vi "Template update scenario templates.vi"(8 "error in (no error)":errorcluster, 9 "ixTemplate (0)":i32, 10 "new name":string, 11 "Connection Refnum":T1) -> (0 "error out":errorcluster, 3 "Connection Refnum":T1)   [LabVIEW 2011]
uses:
  SI.LIB/ODBC/SQL Controls/Connection Refnum.ctl
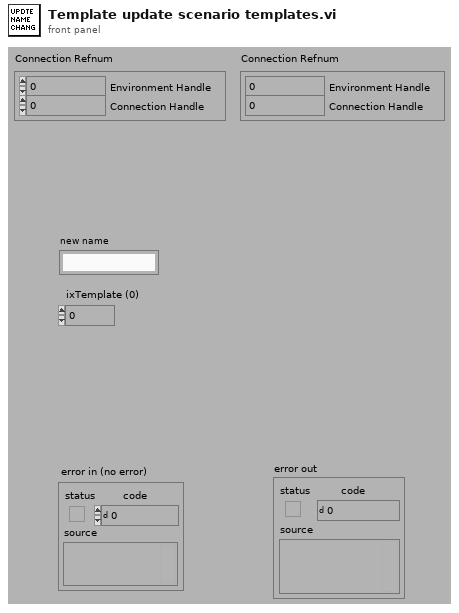
[diagram p1: front panel]
types:
  T1 = typedef "Connection Refnum.ctl" = cluster{"Environment Handle":i32, "Connection Handle":i32}
  T2 = typedef "Template Record.ctl" = cluster{"ixTemplate":i32, "sxTemplateId":string, "sDescription":string, "sCreator":string, "tCreationDate":timestamp, "sModifier":string, "tModifiedDate":timestamp, "sType":string, "sStyle":string, "sFormat":string, "dWidth":dbl, "dHeight":dbl, "sFilename":string, "sScript":string, "sLayout":string, "sEditor":string, "sStyleProcess":string}
  T3 = typedef "Scenario Record.ctl" = cluster{"ixScenario":i32, "tCreated":timestamp, "tModified":timestamp, "sxUsername":string, "sModifiedBy":string, "sxScenarioId":string, "sDescription":string, "sLogic":string, "sResultFieldsCSV":string, "sTemplatesCSV":string, "fAutoRunReports":bool, "fSortByTemplates":bool, "fCombinePDF":bool, "Conditions":T4[]}
  T4 = typedef "Condition Record.ctl" = cluster{"iConditionIndex":i32, "sxFieldId":string, "nOperator":T5, "sMatchValue":string}
  T5 = typedef "Condition Operators.ctl" = enum16{"equal (=)", "not equal (\\u2260)", "less than (<)", "less than or equal (\\u2264)", "greater than (>)", "greater than or equal (\\u2265)", "contains", "does not contain"}
  T6 = typedef "Step Record.ctl" = cluster{"ixStep":i32, "sxSequenceId":string, "sxTestId":string, "iIndex":i32, "iRepeat":i32, "iQuickMode":i32, "sTag":string, "sDatasheetsCSV":string, "bConfiguration":string}
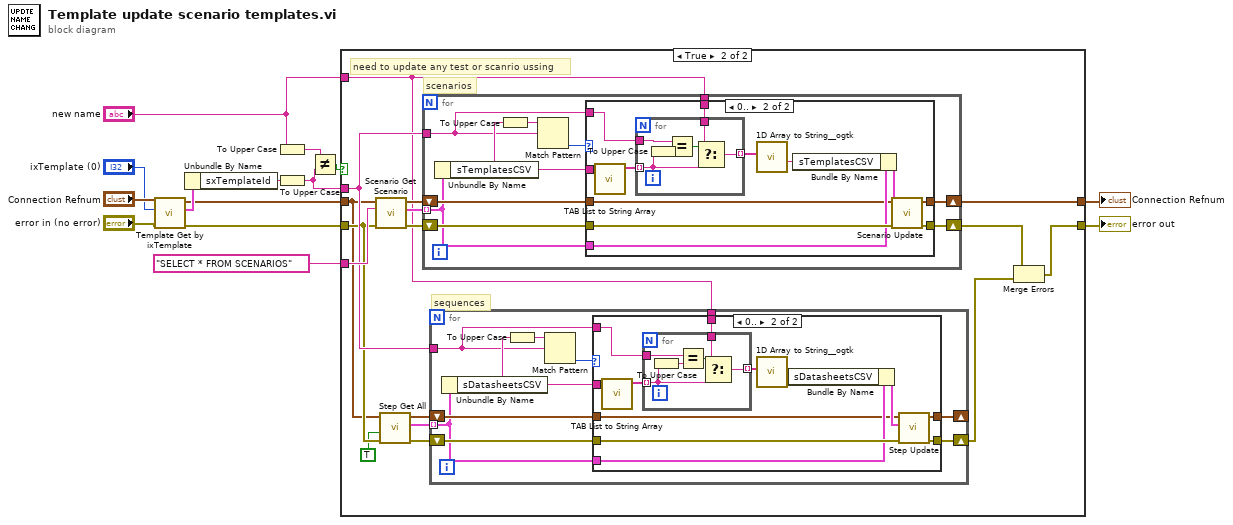
[diagram p0: block diagram]
diagram:
  n1 = call "Template Get by ixTemplate.vi"("error in (no error)"="error in (no error)", "ixTemplate (0)"="ixTemplate (0)", "Connection Refnum"="Connection Refnum") -> ("error out"=w8:errorcluster, "Template Record"=w14:T2, "Connection Refnum"=w6:T1)  [unwired: 6 out]
  n2 = Unbundle By Name(w14) -> ("sxTemplateId"=w13:string)
  n3 = To Upper Case(1:"new name") -> (0:w3:string)
  n4 = To Upper Case(1:w13) -> (0:w2:string)
  n5 = Not Equal?(x=w3, y=w2) -> (x != y?=w9:bool)
  n6 = case shown="True" w9 {
    tunnel: w8 -> [w16 w26]
    tunnel: [w16 w18] -> w7
    tunnel: w6 -> [w15 w21]
    tunnel: [w15 w28] -> w5
    tunnel: "SELECT * FROM SCENARIOS" -> [_ w32]
    tunnel: w2 -> [_ w27]
    tunnel: "new name" -> [_ w22]
    frame False {
      # "same name no update needed"
    }
    frame True {
      # "sequences"
      # "scenarios"
      # "need to update any test or scanrio ussing"
      n7 = call "Scenario Get Scenario.vi"("error in (no error)"=w26, "Query"=w32, "Connection Refnum"=w21) -> ("error out"=w30:errorcluster, "Scenarios"=w31:T3[], "Connection Refnum"=w29:T1)  [unwired: 6 out]
      n8 = call "Step Get All.vi"("error in (no error)"=w26, "All Steps? (f)"=TRUE, "Connection Refnum"=w21) -> ("error out"=w23:errorcluster, "Sequence Steps"=w24:T6[], "Connection Refnum"=w25:T1)  [unwired: 1 in, 5 out]
      n9 = for {
        tunnel: w31 -> [w65] mode=indexing
        shift-right: [w68] -> w20
        shift-left: w30 -> [w69]
        shift-right: [w66] -> w28
        shift-left: w29 -> [w67]
        tunnel: w27 -> [w64]
        tunnel: w22 -> [w63]
        n10 = Unbundle By Name(w65) -> ("sTemplatesCSV"=w72:string)
        n11 = To Upper Case(1:w72) -> (0:w71:string)
        n12 = Match Pattern(string=w71, regular expression=w64) -> (offset past match=w70:i32)  [unwired: 4 out]
        n13 = case shown="0.." w70 {
          tunnel: w72 -> [_ w86]
          tunnel: w69 -> [w74 w85]
          tunnel: [w74 w84] -> w68
          tunnel: w67 -> [w73 w80]
          tunnel: [w73 w83] -> w66
          tunnel: w65 -> [_ w82]
          tunnel: w64 -> [_ w78]
          tunnel: w63 -> [_ w77]
          frame Default {
          }
          frame 0.. {
            n14 = call "TAB List to String Array.vi"("String"=w86) -> ("Array"=w79:string[])  [unwired: 10 out]
            n15 = for {
              tunnel: w79 -> [w90] mode=indexing
              tunnel: w78 -> [w91]
              tunnel: [w89] -> w76 mode=indexing
              tunnel: w77 -> [w88]
              n16 = To Upper Case(1:w90) -> (0:w87:string)
              n17 = Equal?(x=w91, y=w87) -> (x = y?=w92:bool)
              n18 = Select(t=w88, s=w92, f=w90) -> (s? t:f=w89:string)
            }
            n19 = call "1D Array to String__ogtk.vi"("Array of Strings"=w76) -> ("delimited string"=w75:string)  [unwired: 10 in]
            n20 = Bundle By Name(cluster=w82, "sTemplatesCSV"=w75) -> (w81:T3)
            n21 = call "Scenario Update.vi"("error in (no error)"=w85, "Scenario (none)"=w81, "Connection Refnum"=w80) -> ("error out"=w84:errorcluster, "Connection Refnum"=w83:T1)  [unwired: 7 out]
          }
        }
      }
      n22 = for {
        tunnel: w24 -> [w35] mode=indexing
        shift-right: [w38] -> w19
        shift-left: w23 -> [w39]
        shift-right: [w36] -> _
        shift-left: w25 -> [w37]
        tunnel: w27 -> [w34]
        tunnel: w22 -> [w33]
        n23 = Unbundle By Name(w35) -> ("sDatasheetsCSV"=w42:string)
        n24 = To Upper Case(1:w42) -> (0:w41:string)
        n25 = Match Pattern(string=w41, regular expression=w34) -> (offset past match=w40:i32)  [unwired: 4 out]
        n26 = case shown="0.." w40 {
          tunnel: w42 -> [_ w56]
          tunnel: w39 -> [w44 w55]
          tunnel: [w44 w54] -> w38
          tunnel: w37 -> [w43 w50]
          tunnel: [w43 w53] -> w36
          tunnel: w35 -> [_ w52]
          tunnel: w34 -> [_ w48]
          tunnel: w33 -> [_ w47]
          frame Default {
          }
          frame 0.. {
            n27 = call "TAB List to String Array.vi"("String"=w56) -> ("Array"=w49:string[])  [unwired: 10 out]
            n28 = for {
              tunnel: w49 -> [w60] mode=indexing
              tunnel: w48 -> [w61]
              tunnel: [w59] -> w46 mode=indexing
              tunnel: w47 -> [w58]
              n29 = To Upper Case(1:w60) -> (0:w57:string)
              n30 = Equal?(x=w61, y=w57) -> (x = y?=w62:bool)
              n31 = Select(t=w58, s=w62, f=w60) -> (s? t:f=w59:string)
            }
            n32 = call "1D Array to String__ogtk.vi"("Array of Strings"=w46) -> ("delimited string"=w45:string)  [unwired: 10 in]
            n33 = Bundle By Name(cluster=w52, "sDatasheetsCSV"=w45) -> (w51:T6)
            n34 = call "Step Update.vi"("error in (no error)"=w55, "Step Record (empty)"=w51, "Connection Refnum"=w50) -> ("error out"=w54:errorcluster, "Connection Refnum"=w53:T1)  [unwired: 7 out]
          }
        }
      }
      n35 = Merge Errors(w20, w19) -> (w18:errorcluster)
    }
  }
  "error out" <- w7
  "Connection Refnum" <- w5
